vi "GUI FFT panel 2x.vi"(8 "error in":errorcluster, 11 "queue name":string) -> (0 "error out":errorcluster)   [LabVIEW 2020]
doc: "FFT viewer panel. Use 'queue name' to define name of queue with current record information."
uses:
  GUI Waveform Info.ctl
panel:
  out "header path":path
  in  "update":bool
  in  "x-ax ref":string
  in  "ylog":enum16{"Linear", "Log"}(ring) caption="Y-scale"
  in  "xlog":enum16{"Linear", "Log"}(ring) caption="X-scale"
  in  "phase":u16(ring) caption="Channel/phase"
  out "grp I":cluster{"SGL":sgl[], "SGL":sgl[]}(graph)
  out "grp U":cluster{"SGL":sgl[], "SGL":sgl[]}(graph)
  # "Warning: This panel shows FFT spectra only if the algorithm (i) calculates it; (ii) returns it; (iii) qwtb_list.info defines default spectrum quantitites. It will not process waveforms by itself."
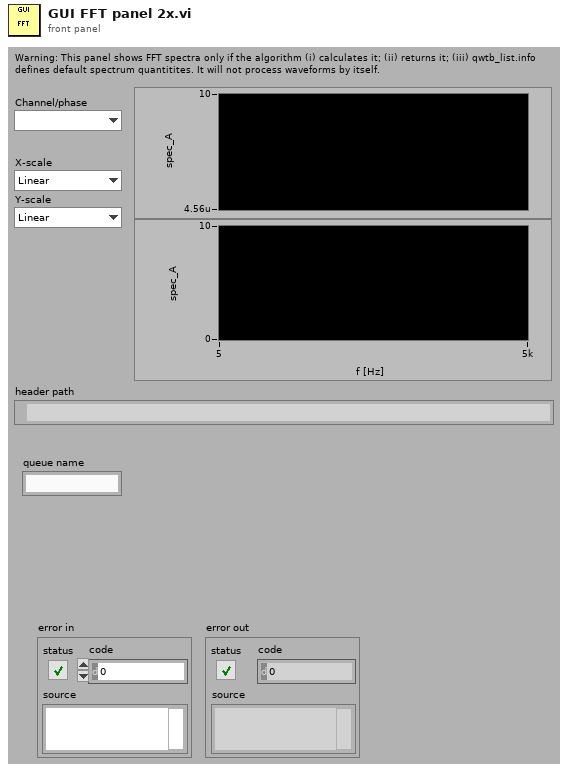
[diagram p1: front panel]
types:
  T1 = typedef "GUI Waveform Info.ctl" = cluster{"header path":path, "group id":i32, "average id":i32, "Time Stamp":timestamp, "max samples":i64, "first sample":i64, "first smpl [%]":dbl, "kill viewer":bool}
  T2 = typedef "Meas Proc QWTB Spectrum Data.ctl" = cluster{"x":sgl[], "y":sgl[], "label":string}
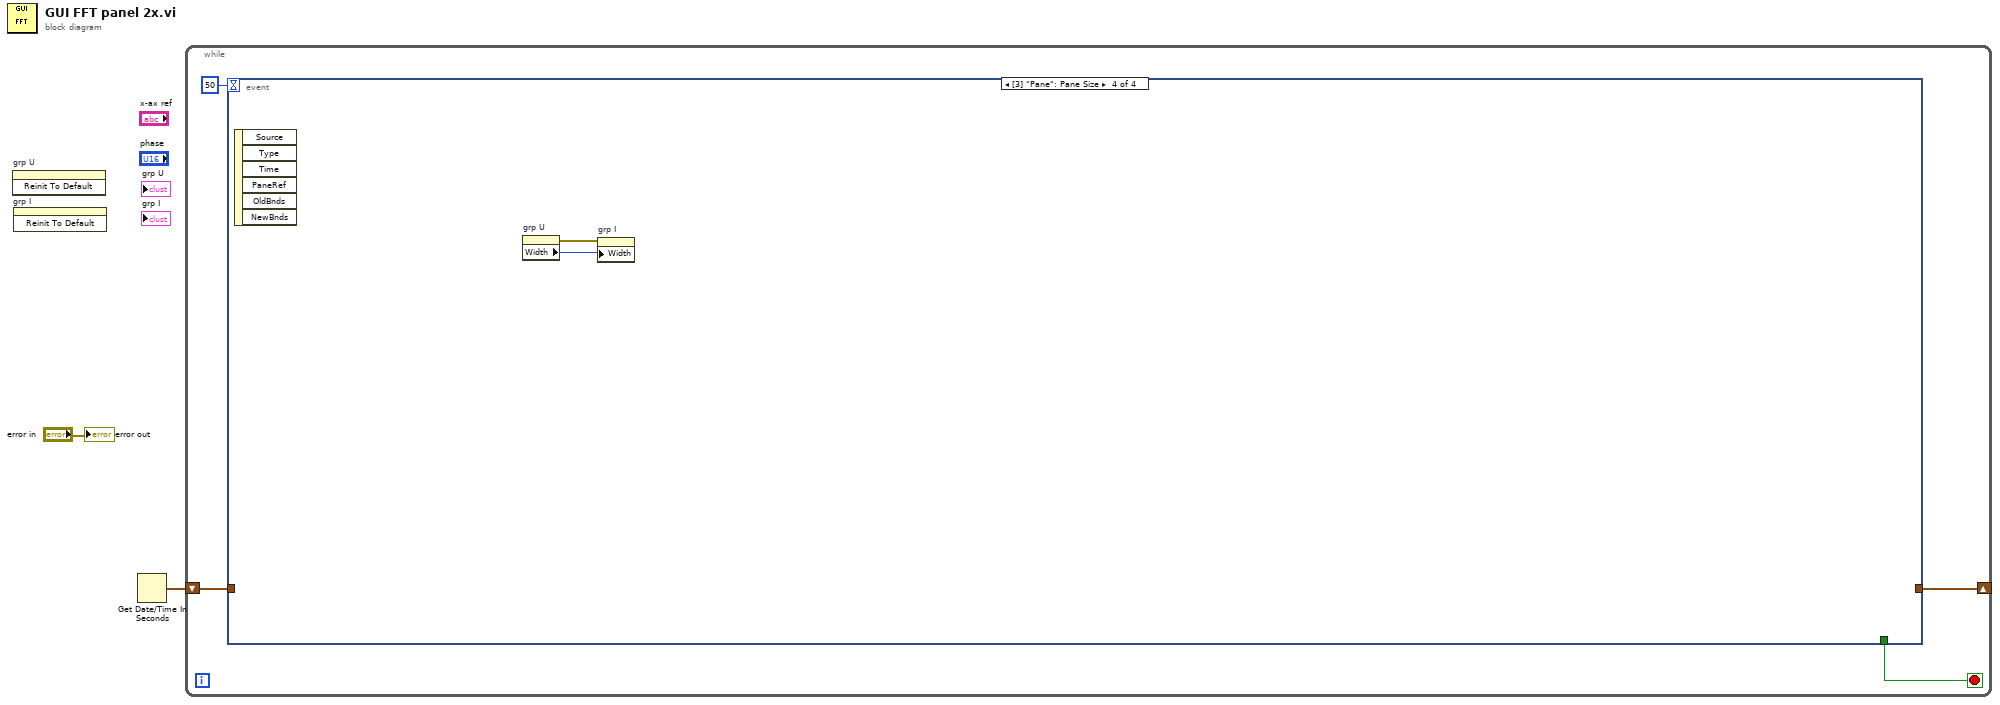
[diagram p0: block diagram]
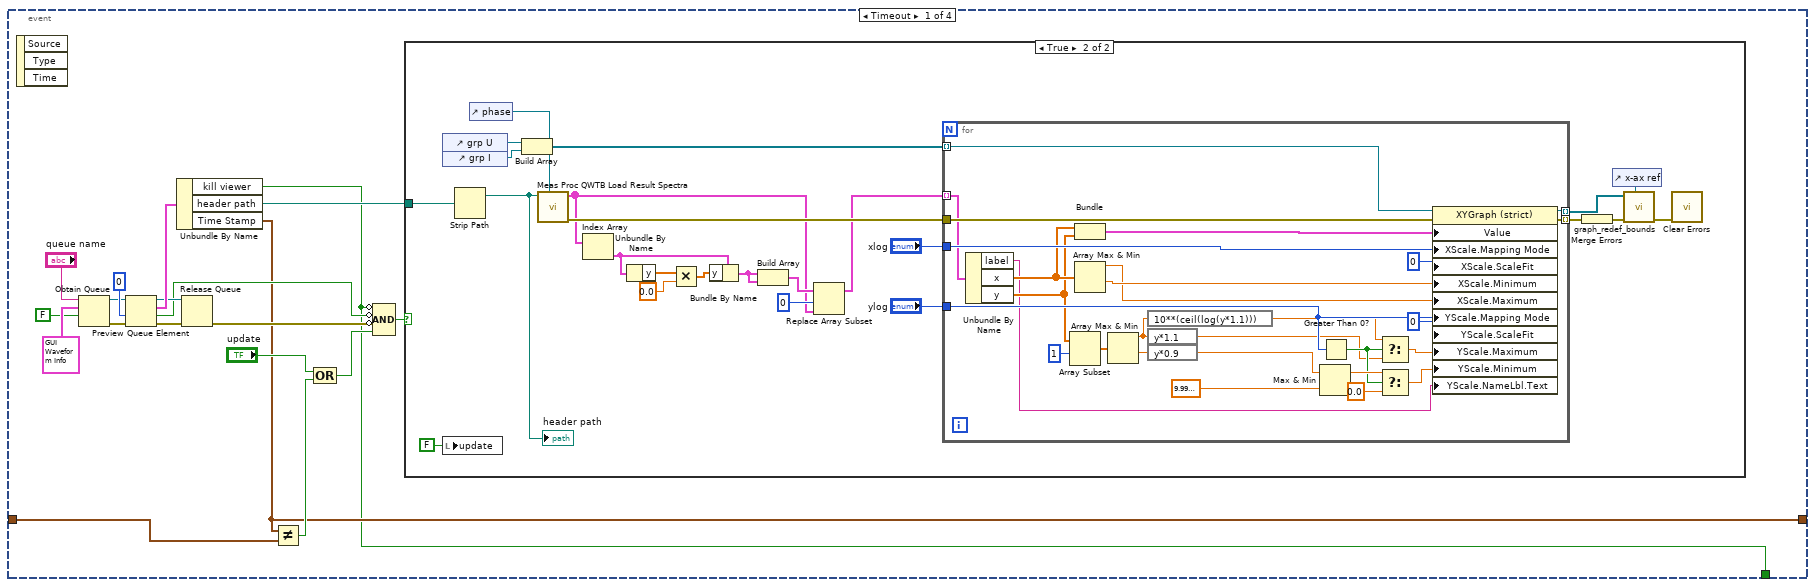
[diagram p2: hidden frame]
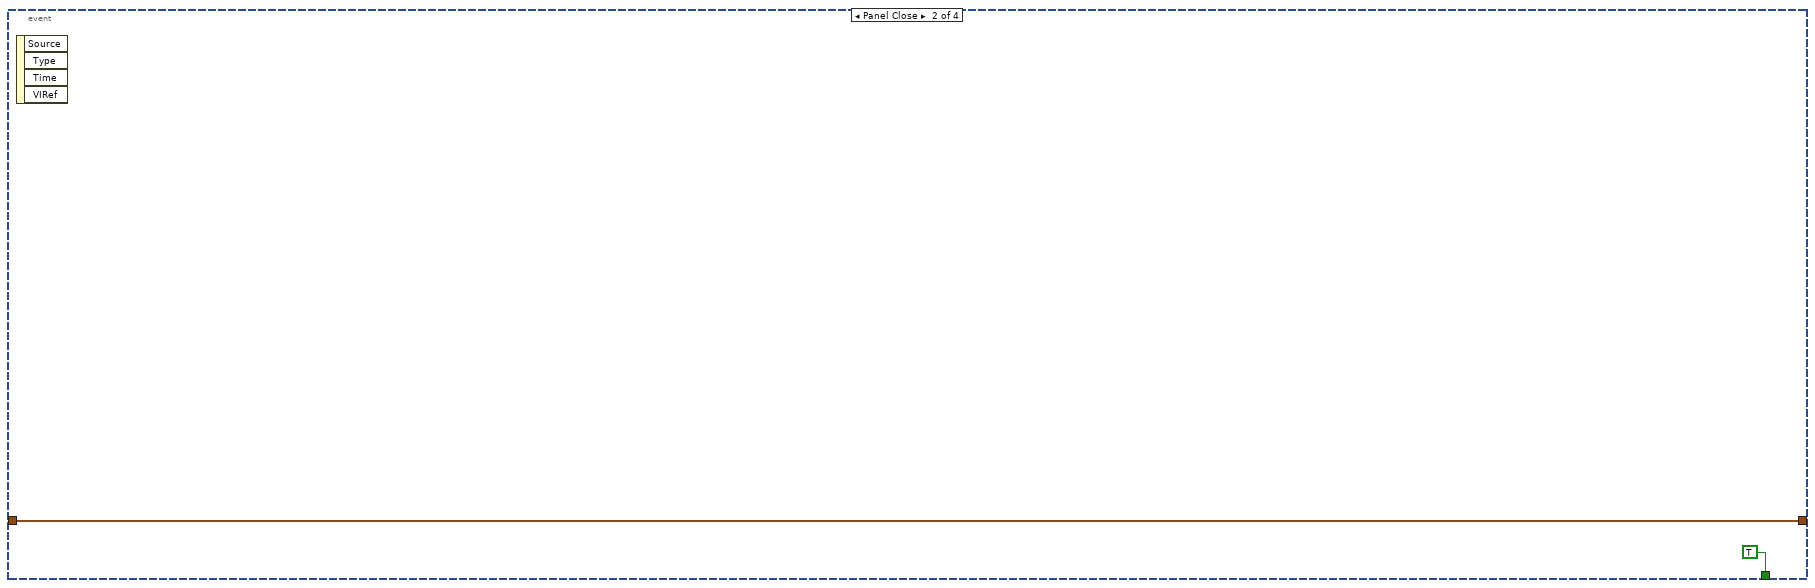
[diagram p4: hidden frame]
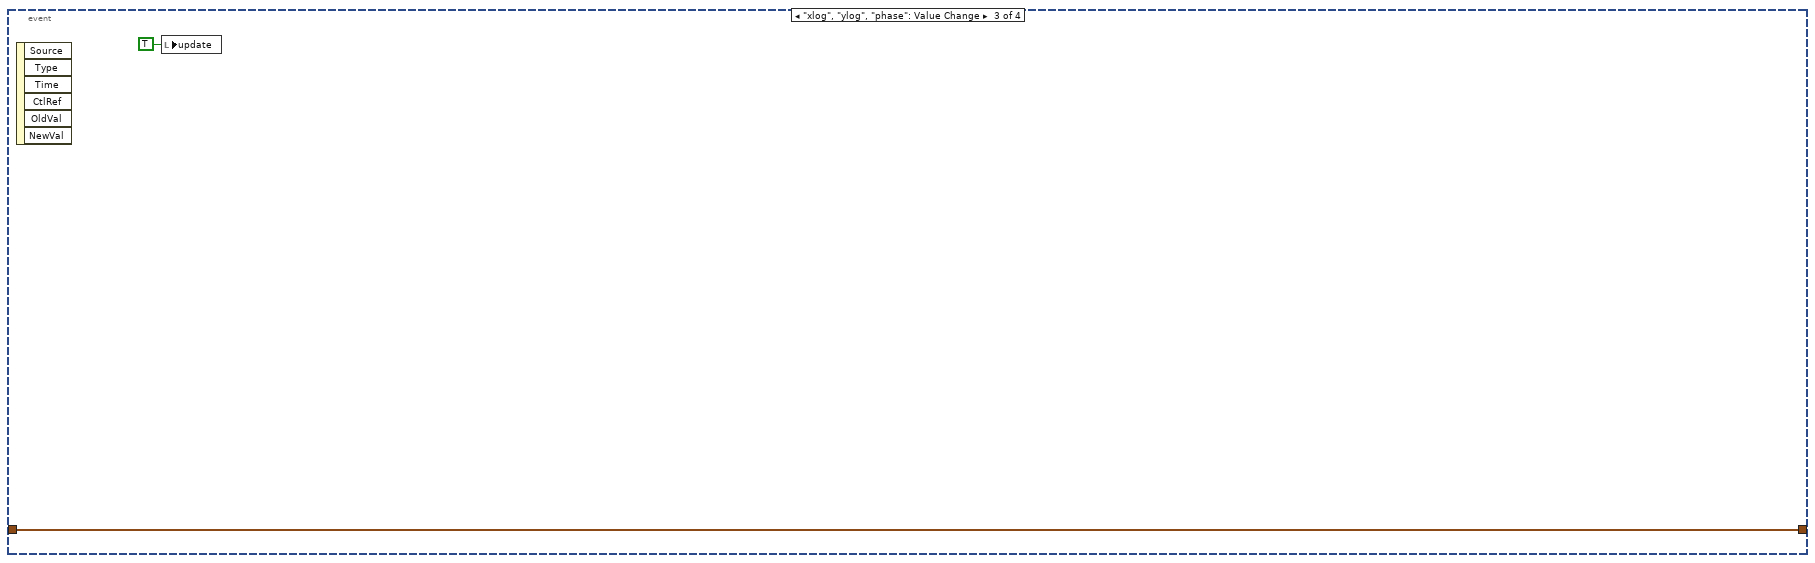
[diagram p5: hidden frame]
diagram:
  n1 = invoke on="grp U" class="XYGraph (strict)" method="Reinit To Default"() -> ()  [unwired: 3 in, 3 out]
  n2 = invoke on="grp I" class="XYGraph (strict)" method="Reinit To Default"() -> ()  [unwired: 3 in, 3 out]
  n3 = Get Date/Time In Seconds() -> (seconds since 1Jan1904=w1:timestamp)
  n4 = while {
    shift-right: [w4] -> _
    shift-left: w1 -> [w5]
    stop <- w6 stop-if-true
    n5 = event shown="[3] \"Pane\": Pane Size" {
      selector: _ -> [_ _ _ _]
      dyn-events: _ -> [_ _ _ _]
      timeout: 50 -> [_ _ _ _]
      tunnel: [w7 TRUE _ _] -> w6
      tunnel: w5 -> [w15 w78 w81 _]
      tunnel: [w9 w78 w81 _] -> w4
      event Timeout {
        n6 = event-data() -> ()  [unwired: 1 in, 3 out]
        n7 = Obtain Queue(name (unnamed)="queue name", element data type=T1 {"header path"=path "", "group id"=0, "average id"=0, "Time Stamp"=timestamp(0 s since 1904-01-01), "max samples"=0, "first sample"=0, "first smpl [%]"=0.0, "kill viewer"=FALSE} ("record info"), create if not found? (T)=FALSE) -> (queue out=w20:refnum<queue>, error out=w19:errorcluster)  [unwired: 2 in, 1 out]
        n8 = Preview Queue Element(queue=w20, timeout in ms (-1)=0, error in (no error)=w19) -> (queue out=w17:refnum<queue>, element=w24:T1, timed out?=w10:bool, error out=w18:errorcluster)
        n9 = Unbundle By Name(w24) -> ("kill viewer"=w7:bool, "header path"=w23:path, "Time Stamp"=w9:timestamp)
        n10 = Release Queue(queue=w17, error in (no error)=w18) -> (error out=w12:errorcluster)  [unwired: 1 in, 2 out]
        n11 = Not Equal?(x=w9, y=w15) -> (x != y?=w14:bool)
        n12 = Compound Arithmetic op=OR("update", w14) -> (w11:bool)
        n13 = Compound Arithmetic op=AND(invert w7, invert w10, invert w12, w11) -> (w13:bool)
        n14 = case shown="True" w13 {
          tunnel: w23 -> [_ w37]
          frame False {
          }
          frame True {
            n15 = control-ref of="grp U"() -> (w48:refnum<vi>)
            n16 = control-ref of="grp I"() -> (w47:refnum<vi>)
            n17 = local write "update"(FALSE ("update")) -> ()
            n18 = Strip Path(path=w37) -> (stripped path=w36:path)  [unwired: 1 out]
            "header path" <- w36
            n19 = control-ref of="phase"() -> (w49:refnum<vi>)
            n20 = Build Array(w48, w47) -> (w45:refnum<vi>[])
            n21 = call "Meas Proc QWTB Load Result Spectra.vi"("phase ref"=w49, "meas root"=w36) -> ("error out"=w46:errorcluster, "graphs"=w31:T2[])  [unwired: 8 in]
            n22 = Index Array(array=w31) -> (element=w30:T2)  [unwired: 1 in]
            n23 = Unbundle By Name(w30) -> ("y"=w29:sgl[])
            n24 = Multiply(x=w29, y=sgl 0.0) -> (x*y=w28:sgl[])
            n25 = Bundle By Name(cluster=w30, "y"=w28) -> (w27:T2)
            n26 = Build Array(w27, w27) -> (w34:T2[])
            n27 = Replace Array Subset(array=w34, new element=w31, index=0) -> (w32:T2[])
            n28 = for {
              tunnel: w46 -> [w77]
              tunnel: w32 -> [w71] mode=indexing
              tunnel: w45 -> [w76] mode=indexing
              tunnel: "xlog" -> [w75]
              tunnel: [w73] -> w43 mode=indexing
              tunnel: [w72] -> w39 mode=indexing
              tunnel: "ylog" -> [w62]
              n29 = Unbundle By Name(w71) -> ("label"=w55:string, "x"=w58:sgl[], "y"=w57:sgl[])
              n30 = Array Subset(array=w57, index=1) -> (w67:sgl[])  [unwired: 1 in]
              n31 = Bundle("x"=w58, "y"=w57) -> (w56:cluster{"x":sgl[], "y":sgl[]})  [unwired: 1 in]
              n32 = Array Max & Min(array=w58) -> (max value=w69:sgl, min value=w70:sgl)  [unwired: 2 out]
              n33 = Array Max & Min(array=w67) -> (max value=w52:sgl, min value=w65:sgl)  [unwired: 2 out]
              n34 = expression code="10**(ceil(log(y*1.1)))"(w52) -> (w51:sgl)
              n35 = expression code="y*1.1"(w52) -> (w53:sgl)
              n36 = expression code="y*0.9"(w65) -> (w64:sgl)
              n37 = Max & Min(x=w64, y=sgl 1e-08) -> (max(x,y)=w61:sgl)  [unwired: 1 out]
              n38 = Greater Than 0?(x=w62) -> (x > 0?=w54:bool)
              n39 = Select(t=w51, s=w54, f=w53) -> (s? t:f=w50:sgl)
              n40 = Select(t=w61, s=w54, f=sgl 0.0) -> (s? t:f=w60:sgl)
              n41 = property class="XYGraph (strict)"(reference=w76, error in=w77, "Value"=w56, "XScale.Mapping Mode"=w75, "XScale.ScaleFit"=u8 0 ("X Scale.Scale Fit"), "XScale.Minimum"=w70, "XScale.Maximum"=w69, "YScale.Mapping Mode"=w62, "YScale.ScaleFit"=u8 0 ("Y Scale.Scale Fit"), "YScale.Maximum"=w50, "YScale.Minimum"=w60, "YScale.NameLbl.Text"=w55) -> (reference out=w72:refnum<vi>, error out=w73:errorcluster)
            }
            n42 = Merge Errors(w43) -> (w41:errorcluster)
            n43 = control-ref of="x-ax ref"() -> (w40:refnum<vi>)
            n44 = call "graph_redef_bounds.vi"("reference"=w40, "error in"=w41, "graph refs in"=w39) -> ("error out"=w38:errorcluster)  [unwired: 7 in, 1 out]
            n45 = call <vilib>:"Clear Errors.vi"("error in (no error)"=w38) -> ()  [unwired: 5 in, 2 out]
          }
        }
      }
      event Panel Close {
        n46 = event-data() -> ()  [unwired: 1 in, 4 out]
      }
      event "xlog", "ylog", "phase": Value Change {
        n47 = event-data() -> ()  [unwired: 1 in, 6 out]
        n48 = local write "update"(TRUE ("update")) -> ()
      }
      event Pane Size {
        n49 = event-data() -> ()  [unwired: 1 in, 6 out]
        n50 = property on="grp U" class="XYGraph (strict)"() -> (error out=w83:errorcluster, "Width"=w82:u32)  [unwired: 2 in, 1 out]
        n51 = property on="grp I" class="XYGraph (strict)"(error in=w83, "Width"=w82) -> ()  [unwired: 1 in, 2 out]
      }
    }
  }
  "error out" <- "error in"
